vi "Save File DOE Save Previous Input Data.vi"(7 "State":enum16{"Write", "Read"}(ring), 8 "error in (no error)":errorcluster, 10 "Appliance Previous Run Path":path=path "C:/GE/Washer DOE", 11 "Appliance Details":T1={"FileVersionInfo"={"FileVersion"="", "ProductName"="", "InternalName"="", "CompanyName"="", "LegalCopyright"="", "FileDescription"=""}, "Dishwasher Info"={"Open Cup Weight (gm):"=0.0, "Auto Cup Weight (gm):"=0.0, "Detergent-Dish:"="", "Inlet Temperature-Dish:"="", "Cycle Mode-Dish:"="", "Unit Control-Dish:"="", "Manufacturer-Dish:"=""}, "Washer Info"={"Hot Water Temperature (Fahrenheit):"="", "Cold Water Temperature (Fahrenheit):"="", "Capacity (cu.ft):"=0.0, "Initial Cloth Weight:"=0.0, "Cloth Lot:"=0, "Model Family:"="", "Program Name:"="", "Cycle Selection:"="", "Wash Temperature:"="", "Rinse Temperature:"="", "Load Size:"=""}, "File Name Output Array"=[], "Calibration Output Array"=[], "Appliance Common"={"Engineer:"="", "Model Number:"="", "Serial Number:"="", "Comments:"="", "Station ID:"="", "Technician:"="", "TR Number:"="", "Lab ID:"="", "Voltage:"="", "Water Pressure (PSI):"="", "Test Date:"="", "Computer Name:"="", "IP Address:"="", "Ambient RH:"="", "Frequency:"="", "Build:"="", "Filename:"="", "Test Type:"="", "Load Run #:"=0, "Ambient Temperature (F):"="", "File Path:"=path "", "Cycles Per Year"=0}, "Water Heater"={"Heating Mode:"=""}, "Dryer"={"Heat Setting:"="", "Washer Water Temperature (60 ± 5°F):"=60, "Water Hardness (PPM):"=17, "Dryness Setting:"="", "Dryer Type:"="", "Exhaust:"="", "Drying Cycle:"="", "Load Type:"="", "Nominal Load Weight"="", "Dryer Initial IMC Data"={"Measured IMC (lbs)"=7.0, "Actual Initial RMC (%)"=7.0, "RMC (Desired %)"=100.0, "Bone Dry Wt(lbs)"=7.0, "Tolerance(%)"=5.0, "Actual Final RMC (%)"=7.0, "CEF (lbf/kWh)"=0.0, "Minimum Weight (lbf)"=0.0, "Average Weight (lbf)"=0.0, "Maximum Weight (lbf)"=0.0, "Measured IMC In Range?"=FALSE, "Moisture Reduction Factor"=55.5, "Field Use Factor"=1.04, "Empty Dryer Cold Weigth"=0.0, "Energy Standard"=enum."D2-Automatic Dryer", "Weight Cloth (lbs)"=0.0, "Relative Moisture Content (%)"=0.0, "Relative Moisture Content - Avg (%)"=0.0}}} {"Dryer"."Dryer Initial IMC Data"."Maximum Weight (lbf)" format="%03_6g"; "Dryer"."Dryer Initial IMC Data"."Average Weight (lbf)" format="%03_6g"; "Dryer"."Dryer Initial IMC Data"."Minimum Weight (lbf)" format="%03_6g"; "Dryer"."Dryer Initial IMC Data"."CEF (lbf/kWh)" format="%03_6g"; "Dryer"."Dryer Initial IMC Data"."Actual Final RMC (%)" format="%03_6g"; "Dryer"."Dryer Initial IMC Data"."Tolerance(%)" format="%0#_6g"; "Dryer"."Dryer Initial IMC Data"."Bone Dry Wt(lbs)" format="%03_6g"; "Dryer"."Dryer Initial IMC Data"."RMC (Desired %)" format="%0#_6g"; "Dryer"."Dryer Initial IMC Data"."Actual Initial RMC (%)" format="%03_6g"; "Dryer"."Dryer Initial IMC Data"."Measured IMC (lbs)" format="%0#_6g"}) -> (0 "error out":errorcluster, 3 "Appliance Details Ouput":T1={"FileVersionInfo"={"FileVersion"="", "ProductName"="", "InternalName"="", "CompanyName"="", "LegalCopyright"="", "FileDescription"=""}, "Dishwasher Info"={"Open Cup Weight (gm):"=0.0, "Auto Cup Weight (gm):"=0.0, "Detergent-Dish:"="", "Inlet Temperature-Dish:"="", "Cycle Mode-Dish:"="", "Unit Control-Dish:"="", "Manufacturer-Dish:"=""}, "Washer Info"={"Hot Water Temperature (Fahrenheit):"="", "Cold Water Temperature (Fahrenheit):"="", "Capacity (cu.ft):"=0.0, "Initial Cloth Weight:"=0.0, "Cloth Lot:"=0, "Model Family:"="", "Program Name:"="", "Cycle Selection:"="", "Wash Temperature:"="", "Rinse Temperature:"="", "Load Size:"=""}, "File Name Output Array"=[], "Calibration Output Array"=[], "Appliance Common"={"Engineer:"="", "Model Number:"="", "Serial Number:"="", "Comments:"="", "Station ID:"="", "Technician:"="", "TR Number:"="", "Lab ID:"="", "Voltage:"="", "Water Pressure (PSI):"="", "Test Date:"="", "Computer Name:"="", "IP Address:"="", "Ambient RH:"="", "Frequency:"="", "Build:"="", "Filename:"="", "Test Type:"="", "Load Run #:"=0, "Ambient Temperature (F):"="", "File Path:"=path "", "Cycles Per Year"=0}, "Water Heater"={"Heating Mode:"=""}, "Dryer"={"Heat Setting:"="", "Washer Water Temperature (60 ± 5°F):"=60, "Water Hardness (PPM):"=17, "Dryness Setting:"="", "Dryer Type:"="", "Exhaust:"="", "Drying Cycle:"="", "Load Type:"="", "Nominal Load Weight"="", "Dryer Initial IMC Data"={"Measured IMC (lbs)"=7.0, "Actual Initial RMC (%)"=7.0, "RMC (Desired %)"=100.0, "Bone Dry Wt(lbs)"=7.0, "Tolerance(%)"=5.0, "Actual Final RMC (%)"=7.0, "CEF (lbf/kWh)"=0.0, "Minimum Weight (lbf)"=0.0, "Average Weight (lbf)"=0.0, "Maximum Weight (lbf)"=0.0, "Measured IMC In Range?"=FALSE, "Moisture Reduction Factor"=55.5, "Field Use Factor"=1.04, "Empty Dryer Cold Weigth"=0.0, "Energy Standard"=enum."D2-Automatic Dryer", "Weight Cloth (lbs)"=0.0, "Relative Moisture Content (%)"=0.0, "Relative Moisture Content - Avg (%)"=0.0}}} {"Dryer"."Dryer Initial IMC Data"."Maximum Weight (lbf)" format="%03_6g"; "Dryer"."Dryer Initial IMC Data"."Average Weight (lbf)" format="%03_6g"; "Dryer"."Dryer Initial IMC Data"."Minimum Weight (lbf)" format="%03_6g"; "Dryer"."Dryer Initial IMC Data"."CEF (lbf/kWh)" format="%03_6g"; "Dryer"."Dryer Initial IMC Data"."Actual Final RMC (%)" format="%03_6g"; "Dryer"."Dryer Initial IMC Data"."Tolerance(%)" format="%0#_6g"; "Dryer"."Dryer Initial IMC Data"."Bone Dry Wt(lbs)" format="%03_6g"; "Dryer"."Dryer Initial IMC Data"."RMC (Desired %)" format="%0#_6g"; "Dryer"."Dryer Initial IMC Data"."Actual Initial RMC (%)" format="%03_6g"; "Dryer"."Dryer Initial IMC Data"."Measured IMC (lbs)" format="%0#_6g"})   [LabVIEW 2018, in "File Setup.lvlib"]
uses:
  File Setup.lvlib
  File Setup (Public)/Type Definition/Save File DISH Dishwasher Details.ctl
  <vilib>/Platform/fileVersionInfo.llb/FileVersionInformation.ctl
  Washer DOE/Type Definitions/DOE Appliance Common.ctl
  Custom Pallet Controls/Custom Pallet String.ctl
  File Setup (Public)/Type Definition/DPT IMC Data.ctl
  Washer DOE/Type Definitions/DOE Dryer Standard.ctl
  <vilib>/Utility/file.llb/Write Delimited Spreadsheet (string).vi
  <vilib>/Utility/file.llb/Read Delimited Spreadsheet (string).vi
panel:
  out "all rows":string[][](array[string])
  out "appended array":string[](array[string])
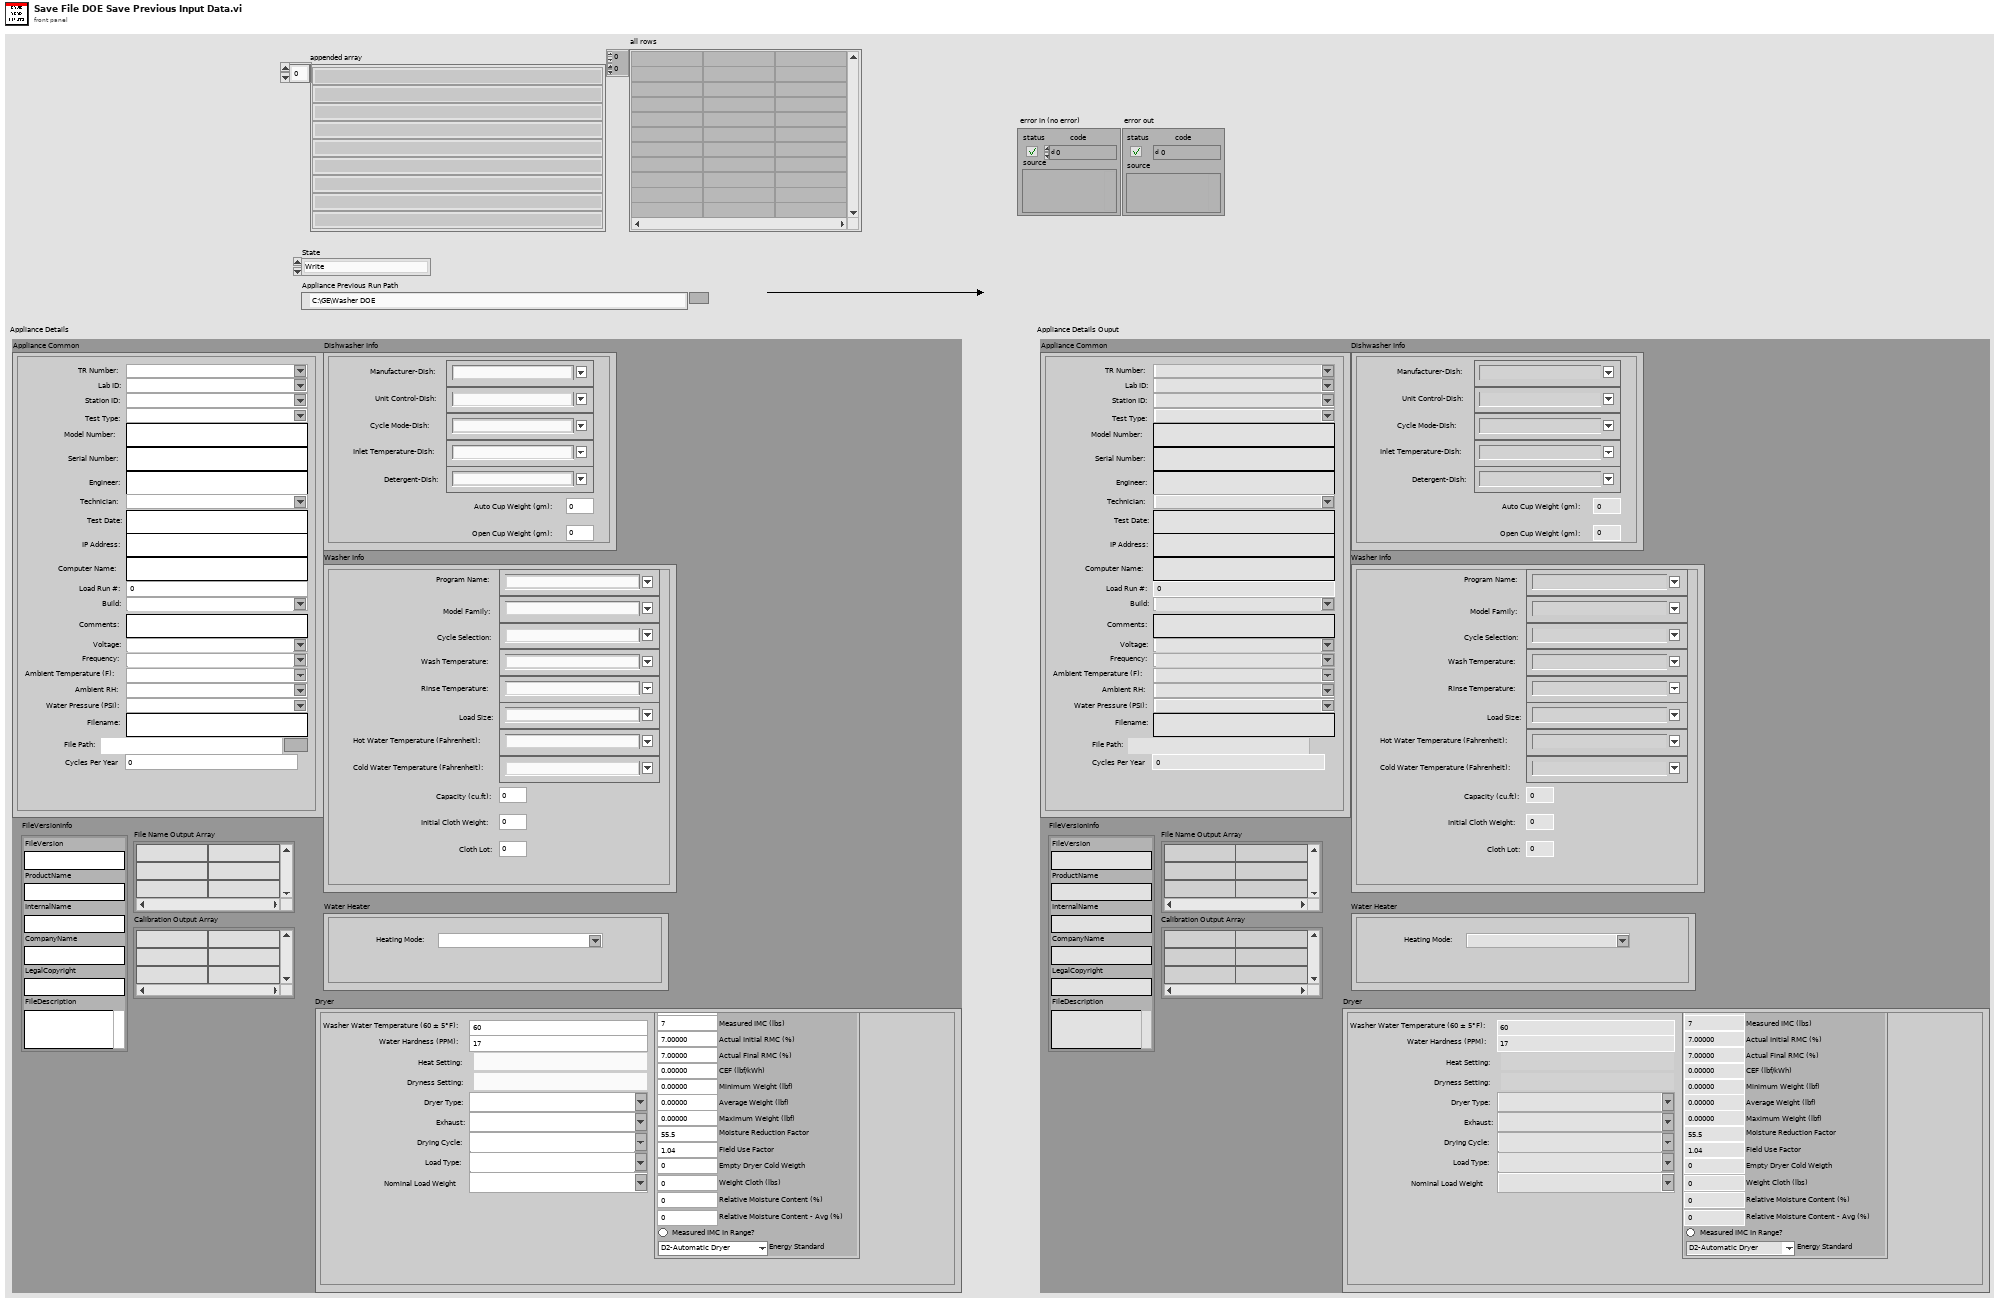
[diagram p1: front panel]
types:
  T1 = typedef "File Setup.lvlib/Save File DISH Dishwasher Details.ctl" = cluster{"FileVersionInfo":T2, "Dishwasher Info":cluster{"Open Cup Weight (gm):":dbl, "Auto Cup Weight (gm):":dbl, "Detergent-Dish:":string, "Inlet Temperature-Dish:":string, "Cycle Mode-Dish:":string, "Unit Control-Dish:":string, "Manufacturer-Dish:":string}, "Washer Info":cluster{"Hot Water Temperature (Fahrenheit):":string, "Cold Water Temperature (Fahrenheit):":string, "Capacity (cu.ft):":dbl, "Initial Cloth Weight:":dbl, "Cloth Lot:":i32, "Model Family:":string, "Program Name:":string, "Cycle Selection:":string, "Wash Temperature:":string, "Rinse Temperature:":string, "Load Size:":string}, "File Name Output Array":string[][], "Calibration Output Array":string[][], "Appliance Common":T3, "Water Heater":cluster{"Heating Mode:":string}, "Dryer":cluster{"Heat Setting:":T4, "Washer Water Temperature (60 ± 5°F):":u16, "Water Hardness (PPM):":u16, "Dryness Setting:":T4, "Dryer Type:":string, "Exhaust:":string, "Drying Cycle:":string, "Load Type:":string, "Nominal Load Weight":string, "Dryer Initial IMC Data":T5}}
  T2 = typedef "FileVersionInformation.ctl" = cluster{"FileVersion":string, "ProductName":string, "InternalName":string, "CompanyName":string, "LegalCopyright":string, "FileDescription":string}
  T3 = typedef "DOE Appliance Common.ctl" = cluster{"Engineer:":string, "Model Number:":string, "Serial Number:":string, "Comments:":string, "Station ID:":string, "Technician:":string, "TR Number:":string, "Lab ID:":string, "Voltage:":string, "Water Pressure (PSI):":string, "Test Date:":string, "Computer Name:":string, "IP Address:":string, "Ambient RH:":string, "Frequency:":string, "Build:":string, "Filename:":string, "Test Type:":string, "Load Run #:":i32, "Ambient Temperature (F):":string, "File Path:":path, "Cycles Per Year":u32}
  T4 = typedef "Custom Pallet String.ctl" = string
  T5 = typedef "DPT IMC Data.ctl" = cluster{"Measured IMC (lbs)":dbl, "Actual Initial RMC (%)":dbl, "RMC (Desired %)":dbl, "Bone Dry Wt(lbs)":dbl, "Tolerance(%)":dbl, "Actual Final RMC (%)":dbl, "CEF (lbf/kWh)":dbl, "Minimum Weight (lbf)":dbl, "Average Weight (lbf)":dbl, "Maximum Weight (lbf)":dbl, "Measured IMC In Range?":bool, "Moisture Reduction Factor":dbl, "Field Use Factor":dbl, "Empty Dryer Cold Weigth":dbl, "Energy Standard":T6, "Weight Cloth (lbs)":dbl, "Relative Moisture Content (%)":dbl, "Relative Moisture Content - Avg (%)":dbl}
  T6 = typedef "DOE Dryer Standard.ctl" = enum16{"D2-Automatic Dryer", "D2-Timer Dryer", "D1-Automatic Dryer", "D1-Timer Dryer", "Other"}
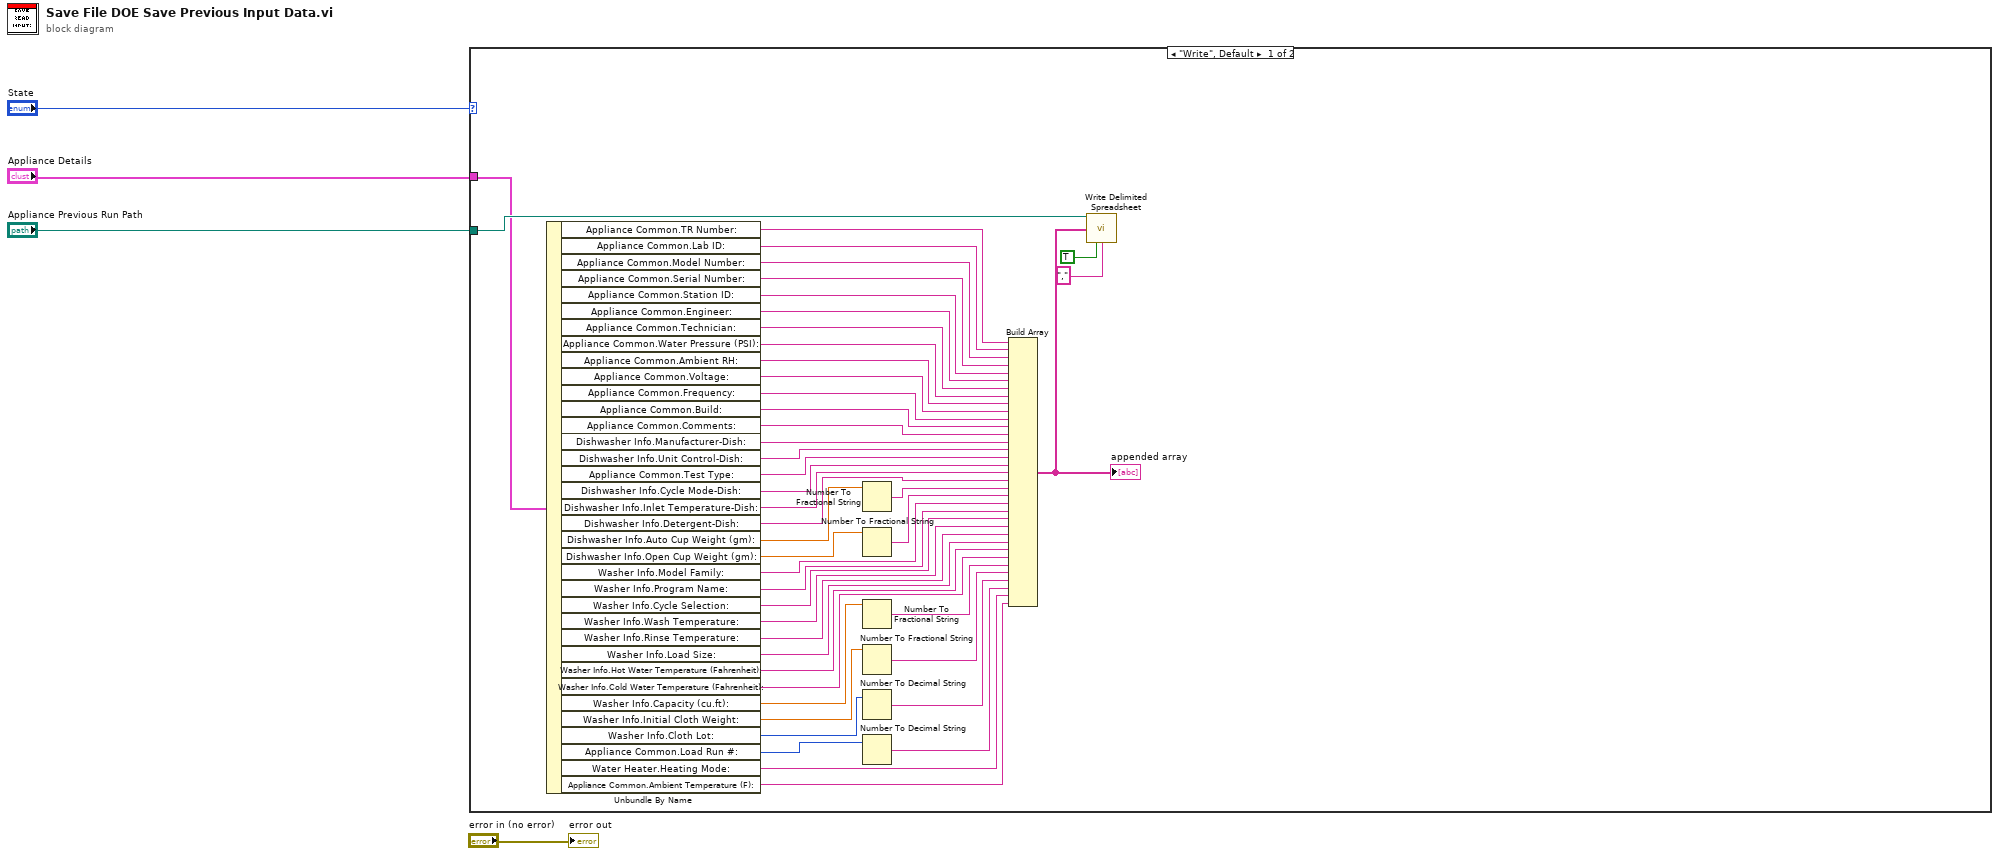
[diagram p0: block diagram]
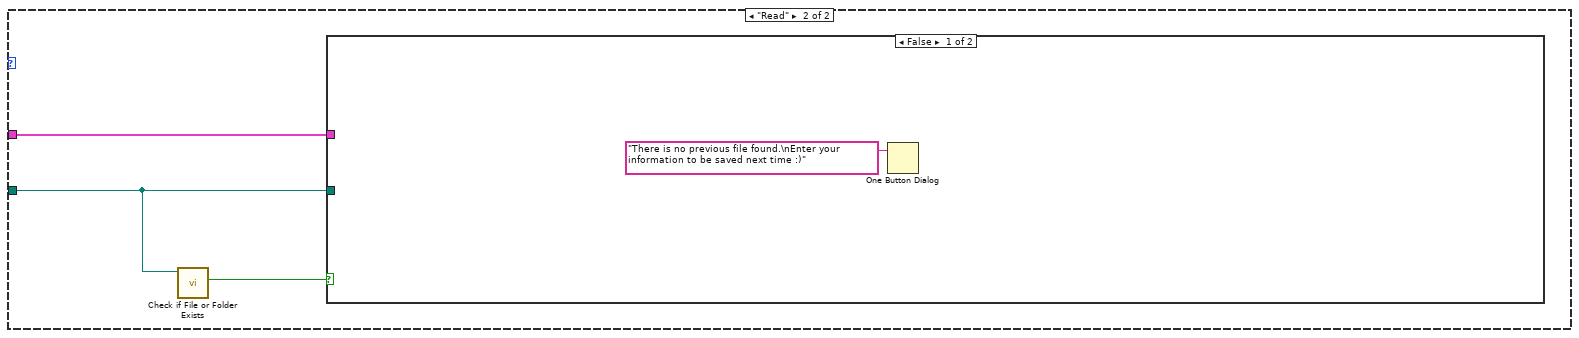
[diagram p2: hidden frame]
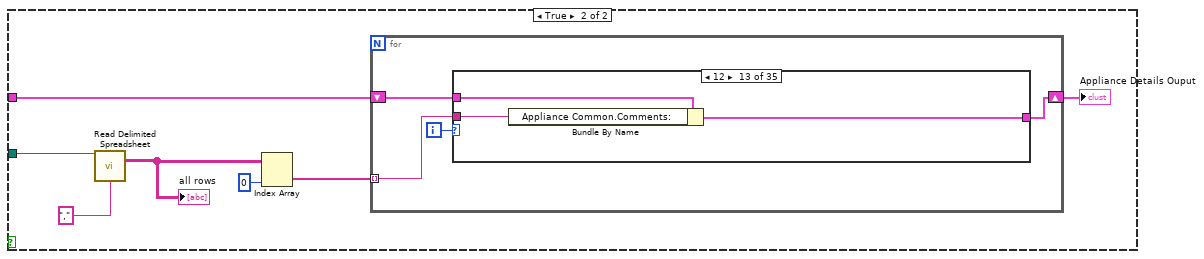
[diagram p3: hidden frame]
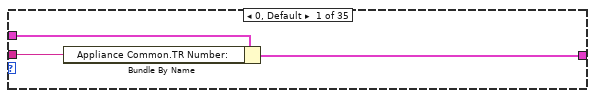
[diagram p4: hidden frame]
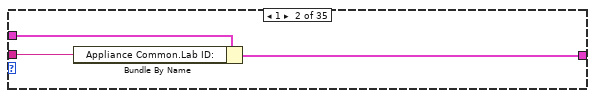
[diagram p5: hidden frame]
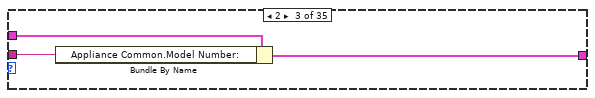
[diagram p6: hidden frame]
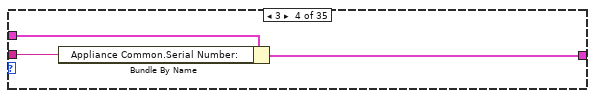
[diagram p7: hidden frame]
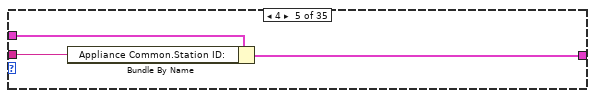
[diagram p8: hidden frame]
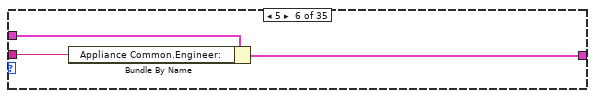
[diagram p9: hidden frame]
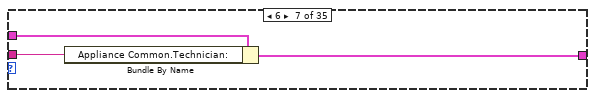
[diagram p10: hidden frame]
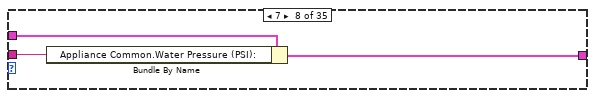
[diagram p11: hidden frame]
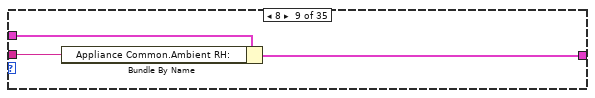
[diagram p12: hidden frame]
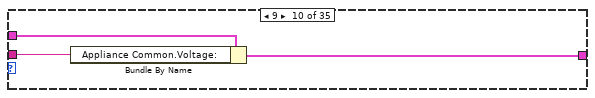
[diagram p13: hidden frame]
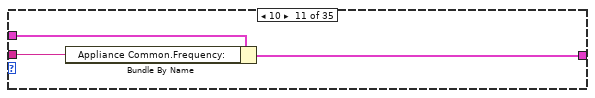
[diagram p14: hidden frame]
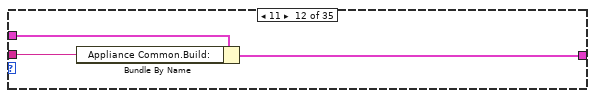
[diagram p15: hidden frame]
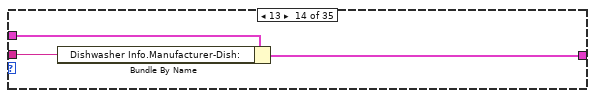
[diagram p16: hidden frame]
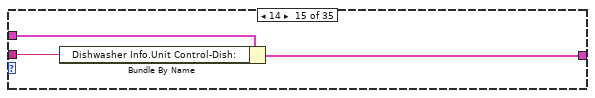
[diagram p17: hidden frame]
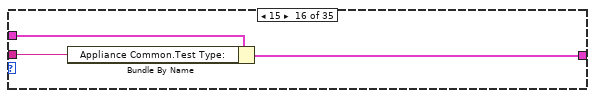
[diagram p18: hidden frame]
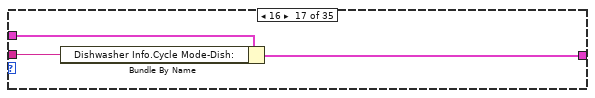
[diagram p19: hidden frame]
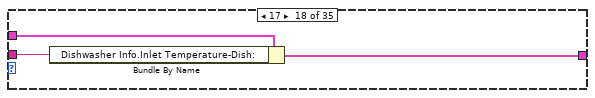
[diagram p20: hidden frame]
diagram:
  n1 = case shown="\"Write\", Default" "State" {
    tunnel: "Appliance Previous Run Path" -> [w11 w52]
    tunnel: "Appliance Details" -> [w8 w53]
    frame "Write", Default {
      n2 = Unbundle By Name(w8) -> ("Appliance Common.TR Number:"=w44:string, "Appliance Common.Lab ID:"=w43:string, "Appliance Common.Model Number:"=w42:string, "Appliance Common.Serial Number:"=w41:string, "Appliance Common.Station ID:"=w40:string, "Appliance Common.Engineer:"=w39:string, "Appliance Common.Technician:"=w38:string, "Appliance Common.Water Pressure (PSI):"=w37:string, "Appliance Common.Ambient RH:"=w36:string, "Appliance Common.Voltage:"=w35:string, "Appliance Common.Frequency:"=w34:string, "Appliance Common.Build:"=w33:string, "Appliance Common.Comments:"=w32:string, "Dishwasher Info.Manufacturer-Dish:"=w31:string, "Dishwasher Info.Unit Control-Dish:"=w30:string, "Appliance Common.Test Type:"=w29:string, "Dishwasher Info.Cycle Mode-Dish:"=w28:string, "Dishwasher Info.Inlet Temperature-Dish:"=w27:string, "Dishwasher Info.Detergent-Dish:"=w26:string, "Dishwasher Info.Auto Cup Weight (gm):"=w47:dbl, "Dishwasher Info.Open Cup Weight (gm):"=w48:dbl, "Washer Info.Model Family:"=w23:string, "Washer Info.Program Name:"=w22:string, "Washer Info.Cycle Selection:"=w21:string, "Washer Info.Wash Temperature:"=w20:string, "Washer Info.Rinse Temperature:"=w19:string, "Washer Info.Load Size:"=w18:string, "Washer Info.Hot Water Temperature (Fahrenheit):"=w17:string, "Washer Info.Cold Water Temperature (Fahrenheit):"=w16:string, "Washer Info.Capacity (cu.ft):"=w50:dbl, "Washer Info.Initial Cloth Weight:"=w49:dbl, "Washer Info.Cloth Lot:"=w46:i32, "Appliance Common.Load Run #:"=w45:i32, "Water Heater.Heating Mode:"=w7:string, "Appliance Common.Ambient Temperature (F):"=w6:string)
      n3 = Number To Fractional String(number=w47) -> (F-format string=w25:string)  [unwired: 3 in]
      n4 = Number To Fractional String(number=w48) -> (F-format string=w24:string)  [unwired: 3 in]
      n5 = Number To Fractional String(number=w50) -> (F-format string=w15:string)  [unwired: 3 in]
      n6 = Number To Fractional String(number=w49) -> (F-format string=w14:string)  [unwired: 3 in]
      n7 = Number To Decimal String(number=w46) -> (decimal integer string=w13:string)  [unwired: 1 in]
      n8 = Number To Decimal String(number=w45) -> (decimal integer string=w12:string)  [unwired: 1 in]
      n9 = Build Array(w44, w43, w42, w41, w40, w39, w38, w37, w36, w35, w34, w33, w32, w31, w30, w29, w28, w27, w26, w25, w24, w23, w22, w21, w20, w19, w18, w17, w16, w15, w14, w13, w12, w7, w6) -> (w5:string[])
      "appended array" <- w5
      n10 = call-poly <vilib>:"Write Delimited Spreadsheet.vi"("file path (dialog if empty)"=w11, "1D data"=w5, "transpose? (no:F)"=TRUE, "delimiter (\\t)"="," ("delimiter (\\t)")) -> ()  [unwired: 10 in, 2 out]
    }
    frame "Read" {
      n11 = call <vilib>:"Check if File or Folder Exists.vi"("path"=w52) -> ("file or folder exists?"=w51:bool)  [unwired: 8 in, 2 out]
      n12 = case shown="False" w51 {
        tunnel: w52 -> [_ w61]
        tunnel: w53 -> [_ w57]
        frame False {
          n13 = One Button Dialog(message="There is no previous file found.\nEnter your information to be saved next time :)") -> ()  [unwired: 1 in, 1 out]
        }
        frame True {
          n14 = call-poly <vilib>:"Read Delimited Spreadsheet.vi"("file path (dialog if empty)"=w61, "delimiter (\\t)"="," ("delimiter (\\t)")) -> ("all rows"=w55:string[][])  [unwired: 8 in, 5 out]
          "all rows" <- w55
          n15 = Index Array(array=w55, index (col)=0 ("disabled index (col)")) -> (element=w58:string[])  [unwired: 1 in]
          n16 = for {
            tunnel: w58 -> [w64] mode=indexing
            shift-right: [w63] -> w56
            shift-left: w57 -> [w62]
            i -> [w65]
            n17 = case shown="12" w65 {
              tunnel: w62 -> [w68 w71 w74 w77 w80 w83 w86 w88 w92 w95 w97 w100 w103 w107 w110 w113 w116 w119 w122 w126 w130 w133 w136 w139 w142 w145 w148 w151 w154 w156 w162 w166 w169 w172 w176]
              tunnel: w64 -> [w67 w70 w72 w75 w78 w81 w84 w87 w90 w93 w96 w99 w102 w105 w108 w111 w114 w117 w120 w124 w128 w131 w134 w137 w140 w143 w146 w149 w152 w158 w160 w164 w170 w171 w174]
              tunnel: [w66 w69 w73 w76 w79 w82 w85 w89 w91 w94 w98 w101 w104 w106 w109 w112 w115 w118 w121 w125 w129 w132 w135 w138 w141 w144 w147 w150 w153 w155 w161 w165 w168 w173 w175] -> w63
              frame 0, Default {
                n18 = Bundle By Name(cluster=w68, "Appliance Common.TR Number:"=w67) -> (w66:T1)
              }
              frame 1 {
                n19 = Bundle By Name(cluster=w71, "Appliance Common.Lab ID:"=w70) -> (w69:T1)
              }
              frame 2 {
                n20 = Bundle By Name(cluster=w74, "Appliance Common.Model Number:"=w72) -> (w73:T1)
              }
              frame 3 {
                n21 = Bundle By Name(cluster=w77, "Appliance Common.Serial Number:"=w75) -> (w76:T1)
              }
              frame 4 {
                n22 = Bundle By Name(cluster=w80, "Appliance Common.Station ID:"=w78) -> (w79:T1)
              }
              frame 5 {
                n23 = Bundle By Name(cluster=w83, "Appliance Common.Engineer:"=w81) -> (w82:T1)
              }
              frame 6 {
                n24 = Bundle By Name(cluster=w86, "Appliance Common.Technician:"=w84) -> (w85:T1)
              }
              frame 7 {
                n25 = Bundle By Name(cluster=w88, "Appliance Common.Water Pressure (PSI):"=w87) -> (w89:T1)
              }
              frame 8 {
                n26 = Bundle By Name(cluster=w92, "Appliance Common.Ambient RH:"=w90) -> (w91:T1)
              }
              frame 9 {
                n27 = Bundle By Name(cluster=w95, "Appliance Common.Voltage:"=w93) -> (w94:T1)
              }
              frame 10 {
                n28 = Bundle By Name(cluster=w97, "Appliance Common.Frequency:"=w96) -> (w98:T1)
              }
              frame 11 {
                n29 = Bundle By Name(cluster=w100, "Appliance Common.Build:"=w99) -> (w101:T1)
              }
              frame 12 {
                n30 = Bundle By Name(cluster=w103, "Appliance Common.Comments:"=w102) -> (w104:T1)
              }
              frame 13 {
                n31 = Bundle By Name(cluster=w107, "Dishwasher Info.Manufacturer-Dish:"=w105) -> (w106:T1)
              }
              frame 14 {
                n32 = Bundle By Name(cluster=w110, "Dishwasher Info.Unit Control-Dish:"=w108) -> (w109:T1)
              }
              frame 15 {
                n33 = Bundle By Name(cluster=w113, "Appliance Common.Test Type:"=w111) -> (w112:T1)
              }
              frame 16 {
                n34 = Bundle By Name(cluster=w116, "Dishwasher Info.Cycle Mode-Dish:"=w114) -> (w115:T1)
              }
              frame 17 {
                n35 = Bundle By Name(cluster=w119, "Dishwasher Info.Inlet Temperature-Dish:"=w117) -> (w118:T1)
              }
              frame 18 {
                n36 = Bundle By Name(cluster=w122, "Dishwasher Info.Detergent-Dish:"=w120) -> (w121:T1)
              }
              frame 19 {
                n37 = Fract/Exp String To Number(string=w124) -> (number=w123:dbl)  [unwired: 3 in, 1 out]
                n38 = Bundle By Name(cluster=w126, "Dishwasher Info.Auto Cup Weight (gm):"=w123) -> (w125:T1)
              }
              frame 20 {
                n39 = Fract/Exp String To Number(string=w128) -> (number=w127:dbl)  [unwired: 3 in, 1 out]
                n40 = Bundle By Name(cluster=w130, "Dishwasher Info.Open Cup Weight (gm):"=w127) -> (w129:T1)
              }
              frame 21 {
                n41 = Bundle By Name(cluster=w133, "Washer Info.Model Family:"=w131) -> (w132:T1)
              }
              frame 22 {
                n42 = Bundle By Name(cluster=w136, "Washer Info.Program Name:"=w134) -> (w135:T1)
              }
              frame 23 {
                n43 = Bundle By Name(cluster=w139, "Washer Info.Cycle Selection:"=w137) -> (w138:T1)
              }
              frame 24 {
                n44 = Bundle By Name(cluster=w142, "Washer Info.Wash Temperature:"=w140) -> (w141:T1)
              }
              frame 25 {
                n45 = Bundle By Name(cluster=w145, "Washer Info.Rinse Temperature:"=w143) -> (w144:T1)
              }
              frame 26 {
                n46 = Bundle By Name(cluster=w148, "Washer Info.Load Size:"=w146) -> (w147:T1)
              }
              frame 27 {
                n47 = Bundle By Name(cluster=w151, "Washer Info.Hot Water Temperature (Fahrenheit):"=w149) -> (w150:T1)
              }
              frame 28 {
                n48 = Bundle By Name(cluster=w154, "Washer Info.Cold Water Temperature (Fahrenheit):"=w152) -> (w153:T1)
              }
              frame 29 {
                n49 = Fract/Exp String To Number(string=w158) -> (number=w157:dbl)  [unwired: 3 in, 1 out]
                n50 = Bundle By Name(cluster=w156, "Washer Info.Capacity (cu.ft):"=w157) -> (w155:T1)
              }
              frame 30 {
                n51 = Fract/Exp String To Number(string=w160) -> (number=w159:dbl)  [unwired: 3 in, 1 out]
                n52 = Bundle By Name(cluster=w162, "Washer Info.Initial Cloth Weight:"=w159) -> (w161:T1)
              }
              frame 31 {
                n53 = Decimal String To Number(string=w164) -> (number=w163:i32)  [unwired: 2 in, 1 out]
                n54 = Bundle By Name(cluster=w166, "Washer Info.Cloth Lot:"=w163) -> (w165:T1)
              }
              frame 32 {
                n55 = Decimal String To Number(string=w170) -> (number=w167:i32)  [unwired: 2 in, 1 out]
                n56 = Bundle By Name(cluster=w169, "Appliance Common.Load Run #:"=w167) -> (w168:T1)
              }
              frame 33 {
                n57 = Bundle By Name(cluster=w172, "Water Heater.Heating Mode:"=w171) -> (w173:T1)
              }
              frame 34 {
                n58 = Bundle By Name(cluster=w176, "Appliance Common.Ambient Temperature (F):"=w174) -> (w175:T1)
              }
            }
          }
          "Appliance Details Ouput" <- w56
        }
      }
    }
  }
  "error out" <- "error in (no error)"
